vi "WK6440B_CommandsGlobal.vi"() -> ()   [LabVIEW 2013, in "WK6440B.lvclass"]
uses:
  WK6440B.lvclass
panel:
  in  "WayneKerr 6440B GPIB Setup":T1={"GPIB address"="23", "Instrument name"="WayneKerr 6440B", "Instrument type"=1, "Command \"Initialise LCR\""=":MEAS:EQU-CCT %s; :MEAS:FREQ %d; :MEAS:LEV %1.2fV; :MEAS; :MEAS:RANGE AUTO; :MEAS:SPEED MED; :MEAS:FUNC:C; :TRIG;", "Command \"OC Trim\""=":CAL:OC-TRIM 3;", "Command \"LCR Readout\""="TRIG;"} {"Instrument type" items=["Supply", "LCR"]}
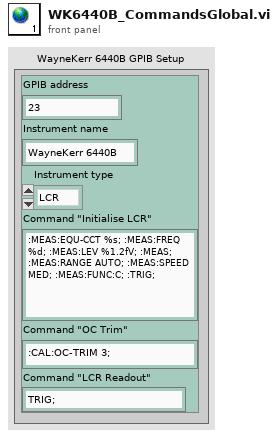
[diagram p1: front panel]
types:
  T1 = cluster{"GPIB address":string, "Instrument name":string, "Instrument type":u16, "Command \"Initialise LCR\"":string, "Command \"OC Trim\"":string, "Command \"LCR Readout\"":string}
diagram:
